vi "ZE_Recorder_ChoseTempConfig.vi"(8 "error in":errorcluster, 11 "Channel Array In":T1 caption="Channel Array" {"Terminal" items=["Default"=-1, "RSE"=10083, "NRSE"=10078, "Differential"=10106, "Pseudodifferential"=12529]}) -> (0 "error out":errorcluster, 2 "keep config":bool, 3 "Channel Array out":T1 caption="Channel Array" {"Terminal" items=["Default"=-1, "RSE"=10083, "NRSE"=10078, "Differential"=10106, "Pseudodifferential"=12529]})   [LabVIEW 2025, in "ZE_Recorder.lvlib"]
uses:
  ZE_Recorder.lvlib
  ZE_Recorder_ChannelCluster.ctl
  ChannelCluster.ctl
  ZE_Recorder_Units.ctl
  Temperature.ctl
  ZE_Recorder_TempChannelAction.ctl
panel:
  # "Connector Pane"
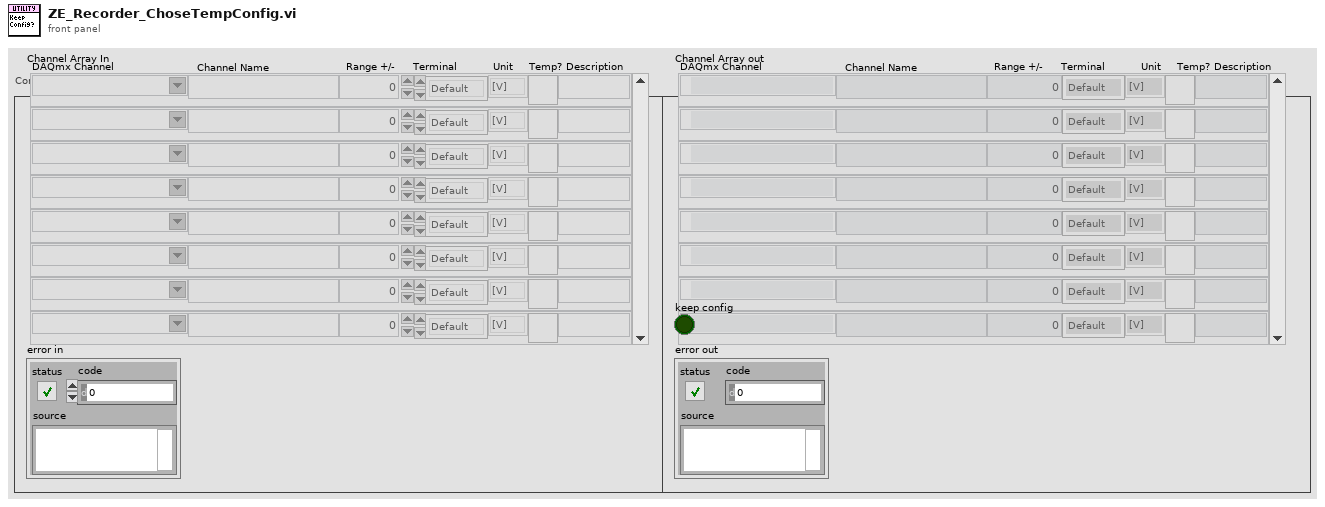
[diagram p1: front panel]
types:
  T1 = typedef "ZE_Recorder.lvlib/ZE_Recorder_ChannelCluster.ctl" = T2[]
  T2 = typedef "ZE_Recorder.lvlib/ChannelCluster.ctl" = cluster{"physical channel":tag, "channel name":string, "Range":dbl, "Terminal":i32, "Unit":T3, "isTemp":T4, "Description":string}
  T3 = typedef "ZE_Recorder.lvlib/ZE_Recorder_Units.ctl" = enum16{"[V]", "[A]", "[F]", "[H]", "[°C]", "[ml/s]", "[m/s]", "[bar]", "[%]", "[N]", "[?]"}
  T4 = typedef "ZE_Recorder.lvlib/Temperature.ctl" = bool
  T5 = typedef "ZE_Recorder.lvlib/ZE_Recorder_TempChannelAction.ctl" = enum16{"Get Channel Configs", "Read Config", "Add Config", "Clear"}
  T6 = typedef "ZE_Recorder.lvlib/ZE_Recorder_TempConfigCluster.ctl" = cluster{"channel name":string, "channel config":T7}
  T7 = typedef "ZE_Recorder.lvlib/ZE_Recorder_TempParam.ctl" = cluster{"ParameterBlock":variant, "TempChannelType":T8}
  T8 = typedef "ZE_Recorder.lvlib/ZE_Recorder_TempType.ctl" = enum16{"none", "Thermocouple", "RTD", "Thermistor VE", "Thermistor CE"}
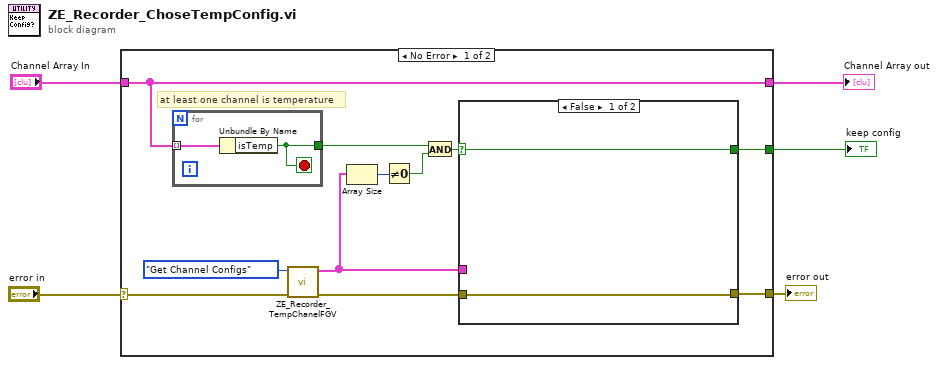
[diagram p0: block diagram]
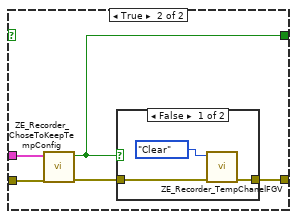
[diagram p2: hidden frame]
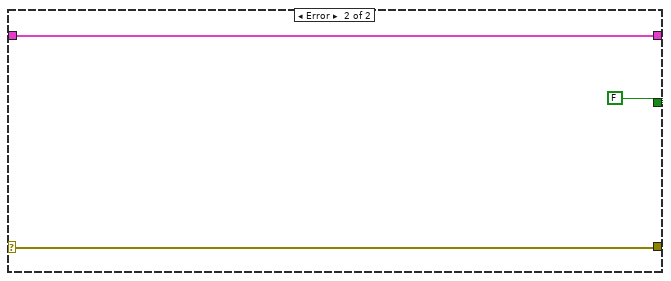
[diagram p4: hidden frame]
diagram:
  n1 = case shown="No Error" "error in" {
    selector: "error in" -> [w14 w32]
    tunnel: "Channel Array In" -> [w16 w31]
    tunnel: [w16 w31] -> w3
    tunnel: [w15 FALSE ("Keep Config?")] -> w2
    tunnel: [w13 w32] -> w1
    frame No Error {
      # "at least one channel is temperature"
      n2 = for {
        tunnel: w16 -> [w29] mode=indexing
        tunnel: [w28] -> w8
        stop <- w28 stop-if-true
        n3 = Unbundle By Name(w29) -> ("isTemp"=w28:T4)
      }
      n4 = call "ZE_Recorder_TempChanelFGV.vi"("error in"=w14, "Action"=ZE_Recorder_TempChannelAction."Get Channel Configs") -> ("error out"=w6:errorcluster, "channel config array"=w11:T6[])  [unwired: 6 in, 2 out]
      n5 = Array Size(array=w11) -> (size(s)=w10:i32)
      n6 = Not Equal To 0?(x=w10) -> (x != 0?=w9:bool)
      n7 = And(x=w8, y=w9) -> (x .and. y?=w7:T4)
      n8 = case shown="False" w7 {
        selector: w7 -> [w18 _]
        tunnel: [w18 w23] -> w15
        tunnel: w6 -> [w17 w19]
        tunnel: [w17 w21] -> w13
        tunnel: w11 -> [_ w20]
        frame False {
        }
        frame True {
          n9 = call "ZE_Recorder_ChoseToKeepTempConfig.vi"("error in"=w19, "channel config array"=w20) -> ("error out"=w22:errorcluster, "Keep Config?"=w23:bool)  [unwired: 8 in]
          n10 = case shown="False" w23 {
            tunnel: w22 -> [w25 w27]
            tunnel: [w26 w27] -> w21
            frame False {
              n11 = call "ZE_Recorder_TempChanelFGV.vi"("error in"=w25, "Action"=ZE_Recorder_TempChannelAction."Clear") -> ("error out"=w26:errorcluster)  [unwired: 6 in, 3 out]
            }
            frame True {
            }
          }
        }
      }
    }
    frame Error {
    }
  }
  "Channel Array out" <- w3
  "keep config" <- w2
  "error out" <- w1
